vi "Actuator selection.vi"(8 "error in (no error)":errorcluster, 11 "RSA in":refnum<class "RSA.lvclass">) -> (0 "error out":errorcluster, 2 "Actuatorout":dbl, 3 "RSA out":refnum<class "RSA.lvclass">)   [LabVIEW 2012, in "RSA.lvclass"]
uses:
  RSA.lvclass
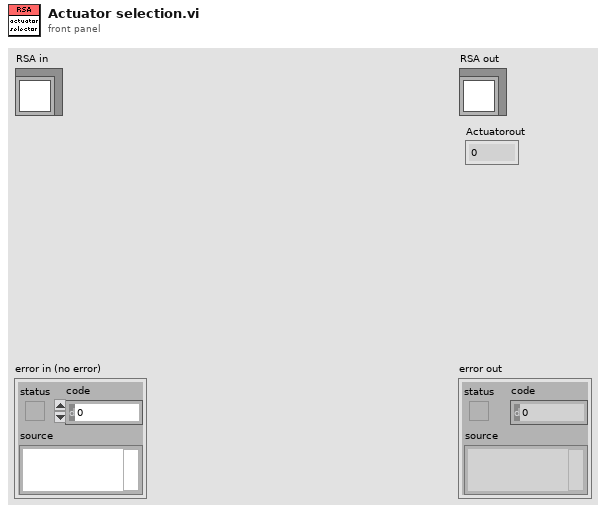
[diagram p1: front panel]
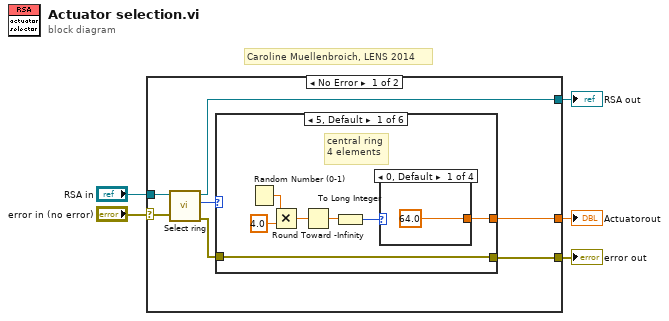
[diagram p0: block diagram]
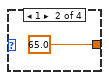
[diagram p2: hidden frame]
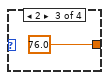
[diagram p3: hidden frame]
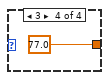
[diagram p4: hidden frame]
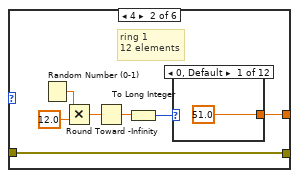
[diagram p5: hidden frame]
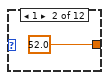
[diagram p6: hidden frame]
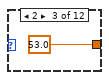
[diagram p7: hidden frame]
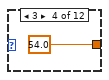
[diagram p8: hidden frame]
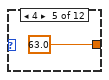
[diagram p9: hidden frame]
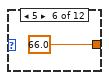
[diagram p10: hidden frame]
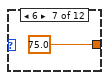
[diagram p11: hidden frame]
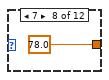
[diagram p12: hidden frame]
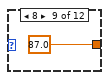
[diagram p13: hidden frame]
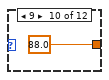
[diagram p14: hidden frame]
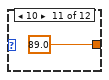
[diagram p15: hidden frame]
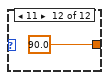
[diagram p16: hidden frame]
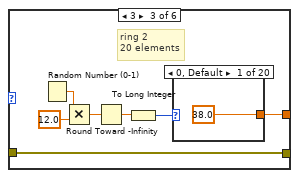
[diagram p17: hidden frame]
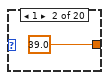
[diagram p18: hidden frame]
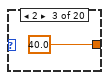
[diagram p19: hidden frame]
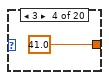
[diagram p20: hidden frame]
diagram:
  # "Caroline Muellenbroich, LENS 2014"
  n1 = case shown="No Error" "error in (no error)" {
    selector: "error in (no error)" -> [w11 w196]
    tunnel: [w8 w196] -> w4
    tunnel: "RSA in" -> [w12 w195]
    tunnel: [w7 w195] -> w2
    tunnel: [w6 _] -> w1
    frame No Error {
      n2 = call-dynamic "Select ring.vi"("error in (no error)"=w11, "RSA in"=w12) -> ("error out"=w9:errorcluster, "Ringnumber"=w10:i32, "RSA out"=w7:refnum<class "RSA.lvclass">)  [unwired: 7 in]
      n3 = case shown="5, Default" w10 {
        tunnel: [w14 w25 w44 w71 w106 w149] -> w6
        tunnel: [w13 w24 w43 w70 w105 w148] -> w8
        tunnel: w9 -> [w13 w24 w43 w70 w105 w148]
        frame 5, Default {
          # "central ring\n4 elements"
          n4 = Random Number (0-1)() -> (number: 0 to 1=w19:dbl)
          n5 = Multiply(x=w19, y=4.0) -> (x*y=w17:dbl)
          n6 = Round Toward -Infinity(1:w17) -> (0:w16:dbl)
          n7 = To Long Integer(number=w16) -> (32bit integer=w15:i32)
          n8 = case shown="0, Default" w15 {
            tunnel: [64.0 ("y") 65.0 ("y") 76.0 ("y") 77.0 ("y")] -> w14
            frame 0, Default {
            }
            frame 1 {
            }
            frame 2 {
            }
            frame 3 {
            }
          }
        }
        frame 4 {
          # "ring 1\n12 elements"
          n9 = Random Number (0-1)() -> (number: 0 to 1=w30:dbl)
          n10 = Multiply(x=w30, y=12.0) -> (x*y=w28:dbl)
          n11 = Round Toward -Infinity(1:w28) -> (0:w27:dbl)
          n12 = To Long Integer(number=w27) -> (32bit integer=w26:i32)
          n13 = case shown="0, Default" w26 {
            tunnel: [51.0 ("y") 52.0 ("y") 53.0 ("y") 54.0 ("y") 63.0 ("y") 66.0 ("y") 75.0 ("y") 78.0 ("y") 87.0 ("y") 88.0 ("y") 89.0 ("y") 90.0 ("y")] -> w25
            frame 0, Default {
            }
            frame 1 {
            }
            frame 2 {
            }
            frame 3 {
            }
            frame 4 {
            }
            frame 5 {
            }
            frame 6 {
            }
            frame 7 {
            }
            frame 8 {
            }
            frame 9 {
            }
            frame 10 {
            }
            frame 11 {
            }
          }
        }
        frame 3 {
          # "ring 2\n20 elements"
          n14 = Random Number (0-1)() -> (number: 0 to 1=w49:dbl)
          n15 = Multiply(x=w49, y=12.0) -> (x*y=w47:dbl)
          n16 = Round Toward -Infinity(1:w47) -> (0:w46:dbl)
          n17 = To Long Integer(number=w46) -> (32bit integer=w45:i32)
          n18 = case shown="0, Default" w45 {
            tunnel: [38.0 ("y") 39.0 ("y") 40.0 ("y") 41.0 ("y") 42.0 ("y") 43.0 ("y") 50.0 ("y") 55.0 ("y") 62.0 ("y") 67.0 ("y") 74.0 ("y") 79.0 ("y") 86.0 ("y") 91.0 ("y") 98.0 ("y") 99.0 ("y") 100.0 ("y") 101.0 ("y") 102.0 ("y") 103.0 ("y")] -> w44
            frame 0, Default {
            }
            frame 1 {
            }
            frame 2 {
            }
            frame 3 {
            }
            frame 4 {
            }
            frame 5 {
            }
            frame 6 {
            }
            frame 7 {
            }
            frame 8 {
            }
            frame 9 {
            }
            frame 10 {
            }
            frame 11 {
            }
            frame 12 {
            }
            frame 13 {
            }
            frame 14 {
            }
            frame 15 {
            }
            frame 16 {
            }
            frame 17 {
            }
            frame 18 {
            }
            frame 19 {
            }
          }
        }
        frame 2 {
          # "ring 3\n28 elements"
          n19 = Random Number (0-1)() -> (number: 0 to 1=w76:dbl)
          n20 = Multiply(x=w76, y=12.0) -> (x*y=w74:dbl)
          n21 = Round Toward -Infinity(1:w74) -> (0:w73:dbl)
          n22 = To Long Integer(number=w73) -> (32bit integer=w72:i32)
          n23 = case shown="0, Default" w72 {
            tunnel: [25.0 ("y") 26.0 ("y") 27.0 ("y") 28.0 ("y") 29.0 ("y") 30.0 ("y") 31.0 ("y") 32.0 ("y") 37.0 ("y") 44.0 ("y") 49.0 ("y") 56.0 ("y") 61.0 ("y") 68.0 ("y") 73.0 ("y") 80.0 ("y") 85.0 ("y") 92.0 ("y") 97.0 ("y") 104.0 ("y") 109.0 ("y") 110.0 ("y") 111.0 ("y") 112.0 ("y") 113.0 ("y") 114.0 ("y") 115.0 ("y") 116.0 ("y")] -> w71
            frame 0, Default {
            }
            frame 1 {
            }
            frame 2 {
            }
            frame 3 {
            }
            frame 4 {
            }
            frame 5 {
            }
            frame 6 {
            }
            frame 7 {
            }
            frame 8 {
            }
            frame 9 {
            }
            frame 10 {
            }
            frame 11 {
            }
            frame 12 {
            }
            frame 13 {
            }
            frame 14 {
            }
            frame 15 {
            }
            frame 16 {
            }
            frame 17 {
            }
            frame 18 {
            }
            frame 19 {
            }
            frame 20 {
            }
            frame 21 {
            }
            frame 22 {
            }
            frame 23 {
            }
            frame 24 {
            }
            frame 25 {
            }
            frame 26 {
            }
            frame 27 {
            }
          }
        }
        frame 1 {
          # "ring 4\n36 elements"
          n24 = Random Number (0-1)() -> (number: 0 to 1=w111:dbl)
          n25 = Multiply(x=w111, y=12.0) -> (x*y=w109:dbl)
          n26 = Round Toward -Infinity(1:w109) -> (0:w108:dbl)
          n27 = To Long Integer(number=w108) -> (32bit integer=w107:i32)
          n28 = case shown="0, Default" w107 {
            tunnel: [12.0 ("y") 13.0 ("y") 14.0 ("y") 15.0 ("y") 16.0 ("y") 17.0 ("y") 18.0 ("y") 19.0 ("y") 20.0 ("y") 21.0 ("y") 24.0 ("y") 33.0 ("y") 36.0 ("y") 45.0 ("y") 48.0 ("y") 57.0 ("y") 60.0 ("y") 69.0 ("y") 72.0 ("y") 81.0 ("y") 84.0 ("y") 93.0 ("y") 96.0 ("y") 105.0 ("y") 108.0 ("y") 117.0 ("y") 120.0 ("y") 121.0 ("y") 122.0 ("y") 123.0 ("y") 124.0 ("y") 125.0 ("y") 126.0 ("y") 127.0 ("y") 128.0 ("y") 129.0 ("y")] -> w106
            frame 0, Default {
            }
            frame 1 {
            }
            frame 2 {
            }
            frame 3 {
            }
            frame 4 {
            }
            frame 5 {
            }
            frame 6 {
            }
            frame 7 {
            }
            frame 8 {
            }
            frame 9 {
            }
            frame 10 {
            }
            frame 11 {
            }
            frame 12 {
            }
            frame 13 {
            }
            frame 14 {
            }
            frame 15 {
            }
            frame 16 {
            }
            frame 17 {
            }
            frame 18 {
            }
            frame 19 {
            }
            frame 20 {
            }
            frame 21 {
            }
            frame 22 {
            }
            frame 23 {
            }
            frame 24 {
            }
            frame 25 {
            }
            frame 26 {
            }
            frame 27 {
            }
            frame 28 {
            }
            frame 29 {
            }
            frame 30 {
            }
            frame 31 {
            }
            frame 32 {
            }
            frame 33 {
            }
            frame 34 {
            }
            frame 35 {
            }
          }
        }
        frame 0 {
          # "ring 5\n40 elements"
          n29 = Random Number (0-1)() -> (number: 0 to 1=w154:dbl)
          n30 = Multiply(x=w154, y=12.0) -> (x*y=w152:dbl)
          n31 = Round Toward -Infinity(1:w152) -> (0:w151:dbl)
          n32 = To Long Integer(number=w151) -> (32bit integer=w150:i32)
          n33 = case shown="39" w150 {
            tunnel: [1.0 ("y") 2.0 ("y") 3.0 ("y") 4.0 ("y") 5.0 ("y") 6.0 ("y") 7.0 ("y") 8.0 ("y") 9.0 ("y") 10.0 ("y") 11.0 ("y") 22.0 ("y") 23.0 ("y") 34.0 ("y") 35.0 ("y") 46.0 ("y") 47.0 ("y") 58.0 ("y") 59.0 ("y") 70.0 ("y") 71.0 ("y") 82.0 ("y") 83.0 ("y") 94.0 ("y") 95.0 ("y") 106.0 ("y") 107.0 ("y") 118.0 ("y") 119.0 ("y") 130.0 ("y") 131.0 ("y") 132.0 ("y") 133.0 ("y") 134.0 ("y") 135.0 ("y") 136.0 ("y") 137.0 ("y") 138.0 ("y") 139.0 ("y") 140.0 ("y")] -> w149
            frame 0, Default {
            }
            frame 1 {
            }
            frame 2 {
            }
            frame 3 {
            }
            frame 4 {
            }
            frame 5 {
            }
            frame 6 {
            }
            frame 7 {
            }
            frame 8 {
            }
            frame 9 {
            }
            frame 10 {
            }
            frame 11 {
            }
            frame 12 {
            }
            frame 13 {
            }
            frame 14 {
            }
            frame 15 {
            }
            frame 16 {
            }
            frame 17 {
            }
            frame 18 {
            }
            frame 19 {
            }
            frame 20 {
            }
            frame 21 {
            }
            frame 22 {
            }
            frame 23 {
            }
            frame 24 {
            }
            frame 25 {
            }
            frame 26 {
            }
            frame 27 {
            }
            frame 28 {
            }
            frame 29 {
            }
            frame 30 {
            }
            frame 31 {
            }
            frame 32 {
            }
            frame 33 {
            }
            frame 34 {
            }
            frame 35 {
            }
            frame 36 {
            }
            frame 37 {
            }
            frame 38 {
            }
            frame 39 {
            }
          }
        }
      }
    }
    frame Error {
    }
  }
  "error out" <- w4
  "RSA out" <- w2
  "Actuatorout" <- w1
